vi "Version.vi"() -> (1 "Build":string, 2 "Version":string)   [LabVIEW 2016]
uses:
  LabVIEW Project API__icon_lib_labview_project_api Folder/LabVIEW Project API__icon_lib_labview_project_api.lvlib
panel:
  out "concatenated string":string
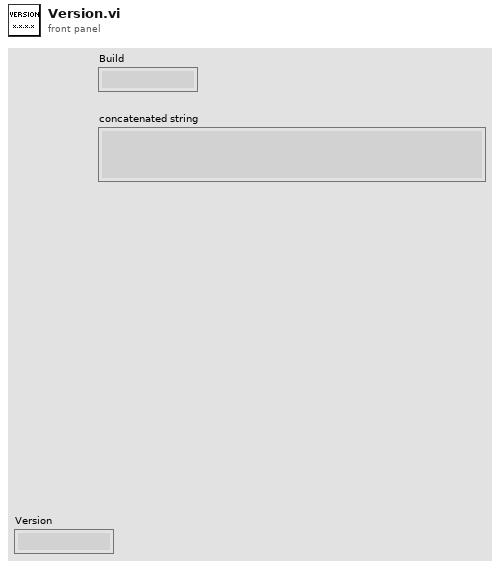
[diagram p1: front panel]
types:
  T1 = enum32{"invalid app kind", "Development System", "Run Time System", "Student Edition", "Embedded LabVIEW", "Evaluation", "Custom"}
  T2 = cluster{"Major":u16, "Minor":u16, "Fix":u16, "Build":u16}
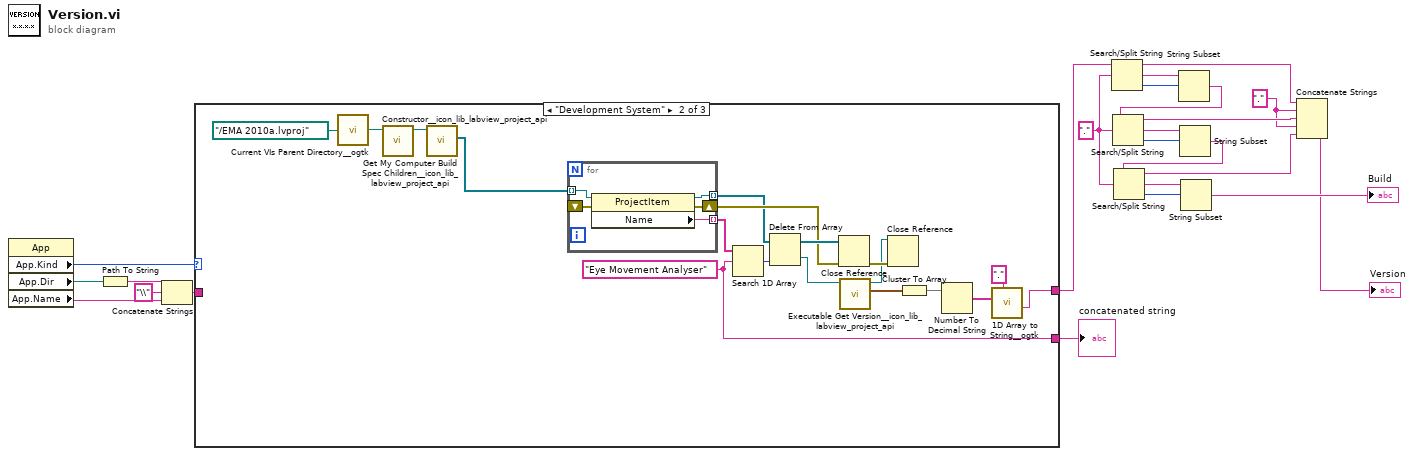
[diagram p0: block diagram]
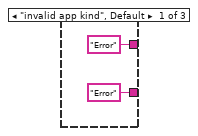
[diagram p2: hidden frame]
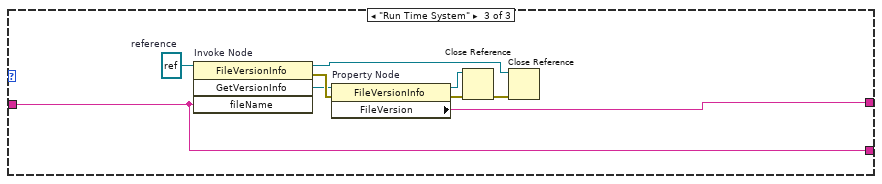
[diagram p3: hidden frame]
diagram:
  w7 = "." ("search string/char (-)")
  w4 = "." ("search string/char (-)")
  n1 = property class="App"() -> ("App.Kind"=w18:T1, "App.Dir"=w23:path, "App.Name"=w22:string)  [unwired: 2 in, 2 out]
  n2 = Path To String(path=w23) -> (string=w21:string)
  n3 = Concatenate Strings(w21, "\\" ("string"), w22) -> (w19:string)
  n4 = case shown="\"Development System\"" w18 {
    tunnel: w19 -> [_ _ w49]
    tunnel: ["Error" ("FileVersion") w26 w50] -> w6
    tunnel: ["Error" ("element") w31 w49] -> w17
    frame "invalid app kind", Default {
    }
    frame "Development System" {
      w31 = "Eye Movement Analyser" ("element")
      n5 = call <userlib>:"Current VIs Parent Directory__ogtk.vi"("Relative path (.)"=path "../EMA 2010a.lvproj") -> ("Parent Directory (+ Relative)"=w43:path)  [unwired: 4 in]
      n6 = call "Constructor__icon_lib_labview_project_api.vi"("Project Path"=w43) -> ("Project Reference"=w41:refnum<vi>)  [unwired: 9 in, 1 out]
      n7 = call "Get My Computer Build Spec Children__icon_lib_labview_project_api.vi"("Project Reference"=w41) -> ("Children[]"=w35:refnum<vi>[])  [unwired: 8 in, 2 out]
      n8 = for {
        shift-right: [w46] -> w39
        shift-left: _ -> [w48]
        tunnel: w35 -> [w47] mode=indexing
        tunnel: [w45] -> w37 mode=indexing
        tunnel: [w44] -> w38 mode=indexing
        n9 = property class="ProjectItem"(reference=w47, error in=w48) -> (reference out=w45:refnum<vi>, error out=w46:errorcluster, "Name"=w44:string)
      }
      n10 = Search 1D Array(1D array=w38, element=w31) -> (index of element=w36:i32)  [unwired: 1 out]
      n11 = Delete From Array(array=w37, index=w36) -> (deleted portion=w34:refnum<vi>, array with subset deleted=w40:refnum<vi>[])  [unwired: 1 in]
      n12 = Close Reference(reference=w40, error in (no error)=w39) -> (error out=w33:errorcluster)
      n13 = call "Executable Get Version__icon_lib_labview_project_api.vi"("Build Spec Reference"=w34) -> ("Version"=w28:T2, "Build Spec Reference Dup"=w32:refnum<vi>)  [unwired: 8 in, 1 out]
      n14 = Close Reference(reference=w32, error in (no error)=w33) -> ()  [unwired: 1 out]
      n15 = Cluster To Array(cluster=w28) -> (array=w27:u16[])
      n16 = Number To Decimal String(number=w27) -> (decimal integer string=w29:string[])  [unwired: 1 out]
      n17 = call <userlib>:"1D Array to String__ogtk.vi"("delimiter (Tab)"=".", "Array of Strings"=w29) -> ("delimited string"=w26:string)  [unwired: 9 out]
    }
    frame "Run Time System" {
      w57 = refnum<k24> refnum  # reference
      n18 = invoke on="Invoke Node" class="FileVersionInfo" method="GetVersionInfo"(reference=w57, "fileName"=w49) -> (reference out=w52:refnum<k24>, error out=w53:errorcluster, "GetVersionInfo"=w51:refnum<k24>)  [unwired: 2 in, 1 out]
      n19 = property on="Property Node" class="FileVersionInfo"(reference=w51, error in=w53) -> (reference out=w54:refnum<k24>, error out=w55:errorcluster, "FileVersion"=w50:string)
      n20 = Close Reference(reference=w54, error in (no error)=w55) -> (error out=w56:errorcluster)
      n21 = Close Reference(reference=w52, error in (no error)=w56) -> ()  [unwired: 1 out]
    }
  }
  "concatenated string" <- w17
  n22 = Search/Split String(string=w6, search string/char (-)=w4) -> (substring before match=w11:string, match + rest of string=w16:string, offset of match=w3:i32)  [unwired: 1 in]
  n23 = String Subset(string=w16, offset (0)=w3) -> (substring=w13:string)  [unwired: 1 in]
  n24 = Search/Split String(string=w13, search string/char (-)=w4) -> (substring before match=w10:string, match + rest of string=w15:string, offset of match=w2:i32)  [unwired: 1 in]
  n25 = String Subset(string=w15, offset (0)=w2) -> (substring=w12:string)  [unwired: 1 in]
  n26 = Search/Split String(string=w12, search string/char (-)=w4) -> (substring before match=w9:string, match + rest of string=w14:string, offset of match=w1:i32)  [unwired: 1 in]
  n27 = String Subset(string=w14, offset (0)=w1) -> (substring=→"Build":string)  [unwired: 1 in]
  n28 = Concatenate Strings(w11, w7, w10, w7, w9) -> (→"Version":string)
